vi "Init Multiple Devices (SubVI).vi"(9 "deviceKey":string) -> (0 "sortie d'erreur":errorcluster, 1 "GetDeviceKeys":string[](array[string]), 2 "Numérique":i32, 3 "Refnum de .NET en sortie":refnum<k24>)   [LabVIEW 2017]
uses:
  dll/CmdLib.dll
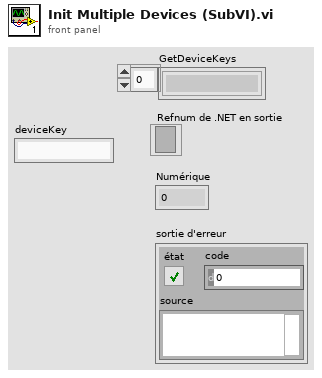
[diagram p1: front panel]
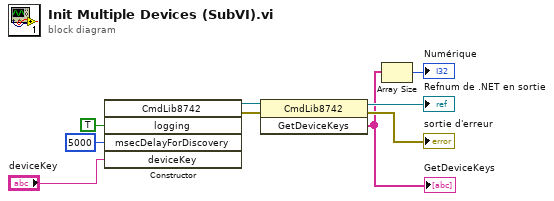
[diagram p0: block diagram]
diagram:
  n1 = constructor class="CmdLib8742"("logging"=TRUE, "msecDelayForDiscovery"=5000, "deviceKey"="deviceKey") -> (reference out=w5:refnum<k24>, error out=w4:errorcluster)  [unwired: 3 in, 4 out]
  n2 = invoke class="CmdLib8742" method="GetDeviceKeys"(reference=w5, error in=w4) -> (reference out=→"Refnum de .NET en sortie":refnum<k24>, error out=→"sortie d'erreur":errorcluster, "GetDeviceKeys"=w6:string[])  [unwired: 1 in]
  "GetDeviceKeys" <- w6
  n3 = Array Size(array=w6) -> (size(s)=→"Numérique":i32)
